vi "Decrement Bearing.vi"(8 "Error In":errorcluster, 10 "Decrement Value":dbl, 11 "Bearing":dbl) -> (0 "Error Out":errorcluster, 3 "New Bearing":dbl)   [LabVIEW 2014]
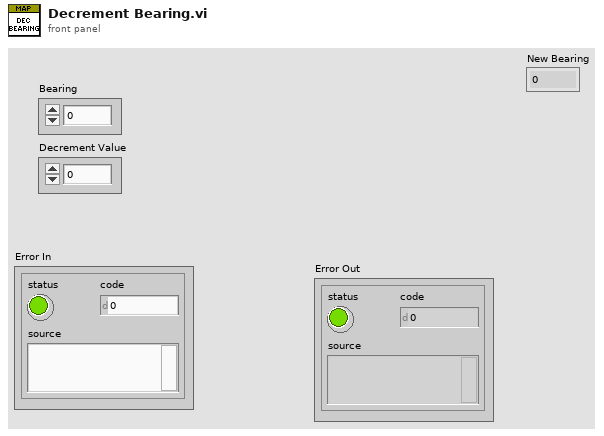
[diagram p1: front panel]
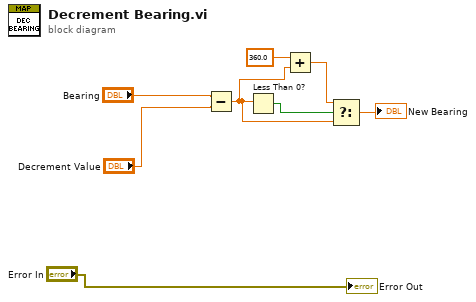
[diagram p0: block diagram]
diagram:
  n1 = Subtract(x="Bearing", y="Decrement Value") -> (x-y=w1:dbl)
  n2 = Less Than 0?(x=w1) -> (x < 0?=w4:bool)
  n3 = Add(x=360.0, y=w1) -> (x+y=w2:dbl)
  n4 = Select(t=w2, s=w4, f=w1) -> (s? t:f=→"New Bearing":dbl)
  "Error Out" <- "Error In"
